vi "pulse length and delay.vi"() -> ()   [LabVIEW 2012]
uses:
  <vilib>/Analysis/NI_AALPro.lvlib
  <vilib>/Analysis/NI_AALBase.lvlib
panel:
  in  "index":i32=625
  out "Sigma":dbl format="%#_3p"
  out "Ch3 Err":dbl format="%_3p"
  out "Ch2 Err":dbl format="%_3p"
  out "Ch1 Err":dbl format="%_3p"
  out "Ch3 Mean":dbl format="%_3p"
  out "Ch2 Mean":dbl format="%_3p"
  out "Ch1 Mean":dbl format="%_3p"
  out "Mean":dbl format="%#_3p"
  in  "Measurement type":i32(ring) items=["Pulse Delay"=1, "Pulse Width"=0]
  out "Sum (%)":dbl format="%#_3g"
  in  "Fit":bool
  in  "Channel4 Threshold Voltage (mV)":i32
  out "Single Count Channel4":dbl format="%#_3p"
  out "Normal part R":dbl format="%#_3g"
  out "Normal part diff":dbl format="%#_3g"
  out "AP part":dbl format="%#_3g"
  out "Normal part Int":dbl format="%#_3f"
  out "Countrate":dbl format="%#_3p"
  out "amplitude":dbl format="%#_3p"
  out "Countrate dinamics":cluster{dbl, dbl, dbl}(graph)
  in  "Histogram Start 1 (ns)":i32=16
  in  "number":i32(ring) items=["Channel3"=2, "Channel2"=1, "Channel1"=0]
  out "Single Count Channel3":dbl format="%#_3p"
  out "Single Count Channel2":dbl format="%#_3p"
  in  "i last":i32
  in  "Reset 1":bool
  in  "Histogram Bin":string(combo)="0"
  out "Waveform Graph 1":cluster{dbl, dbl, dbl[][]}(graph) caption="Waveform Graph"
  out "Single Count Channel1":dbl format="%#_3p"
  out "Exposition time (ms)":i64
  out "Measurement index":i64
  out "Start OK":bool
  in  "Exit":bool
  in  "Channel3 Threshold Voltage (mV)":i32
  in  "Channel2 Threshold Voltage (mV)":i32
  in  "Channel1 Threshold Voltage (mV)":i32 min=0 max=5000 step=10
  in  "Exposition Time (ms)":i64
  # "Current"
  # "Mean"
  # "Err"
  # "Ch1"
  # "Ch2"
  # "Ch3"
  # "Ch4"
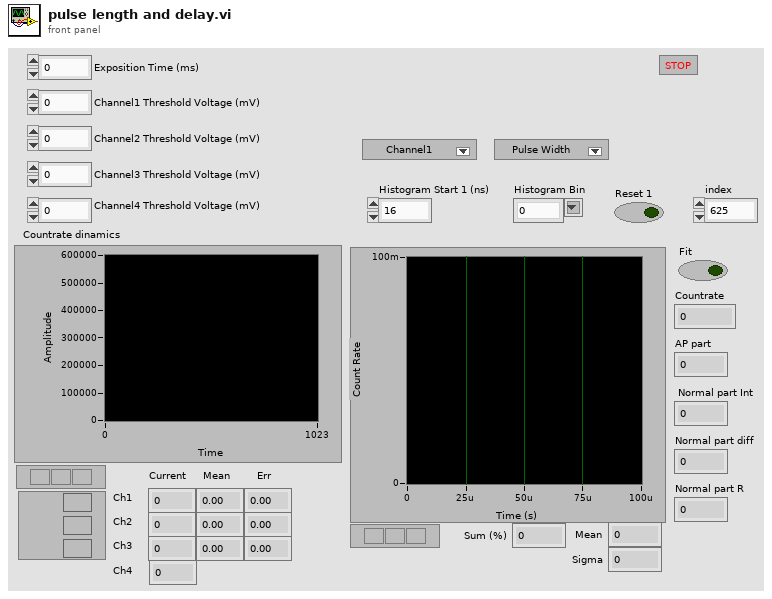
[diagram p1: front panel]
types:
  T1 = cluster{"Channel1":bool, "Channel2":bool, "Channel3":bool, "Channel4":bool}
  T2 = cluster{"[0]":i64, "Channel1 Threshold Voltage (mV)":i32, "Channel1 Pulse Front":string, "Channel2 Threshold Voltage (mV)":i32, "Channel2 Pulse Front":string, "Channel3 Threshold Voltage (mV)":i32, "Channel3 Pulse Front ":string, "Channel4 Threshold Voltage (mV)":i32, "Channel4 Pulse Front ":string, "Single Count Enable":cluster{"Channel1":bool, "Channel2":bool, "Channel3":bool, "Channel4":bool}, "Single Count Max":i32, "Sum Count Enable":cluster{"Channel1":bool, "Channel2":bool, "Channel3":bool, "Channel4":bool}, "Sum Count Max":i32, "Start-Stop1 Multyplex":cluster{"Stop Channel":string, "Start Channel":string}, "Stop Delay 1 (ns)":i16, "Window Length 1 (ns)":i32, "Window Offset 1 (ns) ":i32, "Conditional Correlation 1":string, "Histogram Bin 1":string, "Histogram Start 1 (ns) ":i32, "Start-Stop2 Multyplex ":cluster{"Stop Channel":string, "Start Channel":string}, "Stop Delay 2 (ns)":i16, "Window Length 2 (ns) ":i32, "Window Offset 2 (ns) ":i32, "Conditional Correlation 2":string, "Histogram Bin 2":string, "Histogram Start 2 (ns)  ":i32, "Start-Stop3 Multyplex":cluster{"Stop Channel":string, "Start Channel":string}, "Stop Delay 3 (ns)":i16, "Window Length 3 (ns) ":i32, "Window Offset 3 (ns) ":i32, "Conditional Correlation 3":string, "Histogram Bin 3":string, "Histogram Start 3 (ns) ":i32, "Start-Stop4 Multyplex":cluster{"Stop Channel":string, "Start Channel":string}, "Stop Delay 4 (ns)":i16, "Window Length 4 (ns)  ":i32, "Window Offset 4 (ns) ":i32, "Conditional Correlation 4":string, "Histogram Bin 4":string, "Histogram Start 4 (ns)  ":i32, "Coincidence Count Enable":cluster{"Start-Stop1":bool, "Start-Stop2":bool, "Start-Stop3":bool, "Start-Stop4":bool}, "Coincidence Count Max":i32, "Coincidence Sum Enable":cluster{"Start-Stop1":bool, "Start-Stop2":bool, "Start-Stop3":bool, "Start-Stop4":bool}, "Coincidence Sum Max":i32, "Output Channel Enable":cluster{"Channel1":bool, "Channel2":bool, "Channel3":bool, "Channel4":bool}, "Output Channel Inversion":cluster{"Channel1":bool, "Channel2":bool, "Channel3":bool, "Channel4":bool, "Output":bool}}
  T3 = cluster{"Going":bool, "Iinterrupted":bool, "Timer stop":bool, "Single count stop Ch1":bool, "Single count stop Ch2":bool, "Single count stop Ch3":bool, "Single count stop Ch4":bool, "Sum count stop":bool, "Coincidence count stop SS1":bool, "Coincidence count stop SS2":bool, "Coincidence count stop SS3":bool, "Coincidence count stop SS4":bool, "Coincidence sum count stop":bool, "Reserved":bool, "Correlator is not initialised":bool, "Internal error":bool}
  T4 = cluster{"Measurement index":i64, "Exposition time (ms)":i64, "Single Count Channel1":i64, "Single Count Channel2":i64, "Single Count Channel3":i64, "Single Count Channel4":i64, "Sum Single Count":i64, "Coincidence Count SS1":i64, "Coincidence Count SS2":i64, "Coincidence Count SS4":i64, "Coincidence Count SS5":i64, "Sum Coincidence Count":i64}
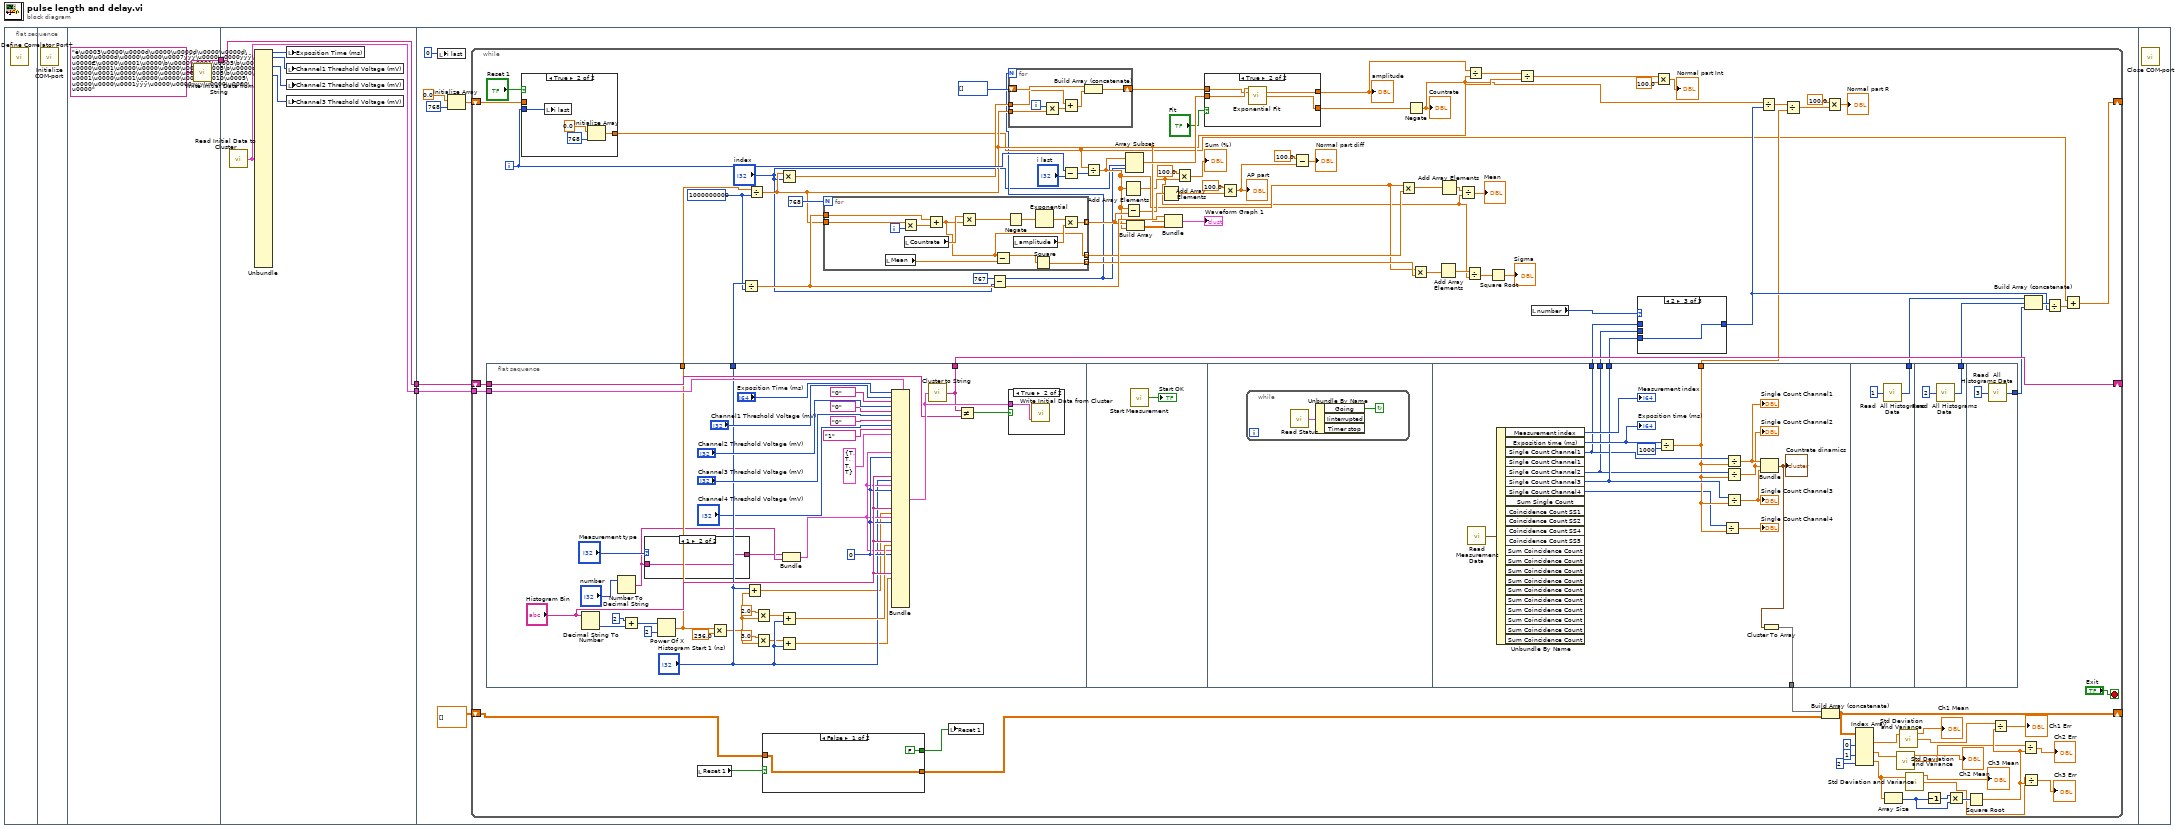
[diagram p0: block diagram]
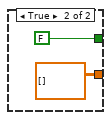
[diagram p2: hidden frame]
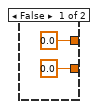
[diagram p3: hidden frame]
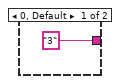
[diagram p7: hidden frame]
diagram:
  n1 = flat-sequence {
    tunnel: [w4] -> w1
    tunnel: [w10] -> w3
    tunnel: [w5] -> w2
    tunnel: w1 -> [w5]
    tunnel: w3 -> [w17]
    tunnel: w2 -> [w13]
    frame #0 {
      n2 = call "Define Correlator Port+.vi"() -> ()  [unwired: 3 in]
    }
    frame #1 {
      n3 = call "Initialize COM-port.vi"() -> ()  [unwired: 4 in]
    }
    frame #2 {
      w4 = "è\u0003\u0000\u0000d\u0000\u0000d\u0000\u0000d\u0000\u0000d\u0000\u0000\u0007ÿÿÿ\u0000\u0000ÿÿÿ\u0000€\u0000\u0001\u0000\b\u0000\u0001\u0005\b\u0000‘\u0000\u0001\u0000\u0000\u0000\u0002\u0005\b\u0000¢\u0000\u0001\u0000\u0000\u0000\u0004\u0005\b\u0000\u0001\u0000\u0001\u0000\u0000\u0000\u0010\u0005\u0000\u0000\u0001ÿÿÿ\u0000\u0000ÿÿÿ\u0000\u0000\u0000" ("string")
      n4 = call "Write Initial Data from String.vi"("Data"=w4) -> ()  [unwired: 1 out]
    }
    frame #3 {
      n5 = call "Read Initial Data to Cluster.vi"() -> ("Correlator Initial Data 2"=w10:T2)  [unwired: 2 in]
      n6 = Unbundle(w10) -> ("[0]"=w9:i64, "Channel1 Threshold Voltage (mV)"=w8:i32, "Channel2 Threshold Voltage (mV)"=w7:i32, "Channel3 Threshold Voltage (mV)"=w6:i32)  [unwired: 43 out]
      n7 = local write "Exposition Time (ms)"(w9) -> ()
      n8 = local write "Channel1 Threshold Voltage (mV)"(w8) -> ()
      n9 = local write "Channel2 Threshold Voltage (mV)"(w7) -> ()
      n10 = local write "Channel3 Threshold Voltage (mV)"(w6) -> ()
    }
    frame #4 {
      n11 = local write "i last"(0 ("i last")) -> ()
      n12 = Initialize Array(0.0 ("element"), 768 ("dimension size")) -> (w14:dbl[])
      n13 = while {
        tunnel: w17 -> [w110]
        shift-right: [w104] -> _
        shift-left: w14 -> [w102]
        shift-right: [w108] -> _
        shift-left: w13 -> [w107]
        shift-right: [w50] -> _
        shift-left: dbl[][] [] -> [w40]
        i -> [w100]
        stop <- "Exit" stop-if-true
        w105 = 1000000000 ("y")
        n14 = flat-sequence {
          tunnel: w110 -> [w182]
          tunnel: ["Histogram Start 1 (ns)"] -> w106
          tunnel: [w175] -> w108
          tunnel: w107 -> [w177]
          tunnel: [w167] -> w88
          tunnel: [w202] -> w91
          tunnel: [w204] -> w90
          tunnel: [w203] -> w92
          tunnel: [w197] -> w63
          tunnel: [w194] -> w51
          tunnel: [w209] -> w97
          tunnel: [w211] -> w95
          tunnel: [w213] -> w94
          frame #0 {
            w165 = i16 0 ("Stop Delay1  (ns)")
            n15 = Decimal String To Number(string="Histogram Bin") -> (number=w173:i32)  [unwired: 2 in, 1 out]
            n16 = Number To Decimal String(number="number") -> (decimal integer string=w152:string)  [unwired: 1 in]
            n17 = Add(x=2, y=w173) -> (x+y=w172:i32)
            n18 = case shown="1" "Measurement type" {
              tunnel: w152 -> [_ w189]
              tunnel: ["3" ("decimal integer string") w189] -> w151
              frame 0, Default {
              }
              frame 1 {
              }
            }
            n19 = Power Of X(1:i8 2 ("x"), 2:w172) -> (0:w167:dbl)
            n20 = Multiply(x=w167, y=256.0) -> (x*y=w161:dbl)
            n21 = Add(x="Histogram Start 1 (ns)", y=w161) -> (x+y=w156:dbl)
            n22 = Multiply(x=2.0, y=w161) -> (x*y=w160:dbl)
            n23 = Multiply(x=3.0, y=w161) -> (x*y=w158:dbl)
            n24 = Add(x=w160, y="Histogram Start 1 (ns)") -> (x+y=w168:dbl)
            n25 = Add(x=w158, y="Histogram Start 1 (ns)") -> (x+y=w162:dbl)
            n26 = Bundle("decimal integer string"=w151, w152) -> (w164:cluster{"decimal integer string":string, string})  [unwired: 1 in]
            n27 = Bundle(cluster=w182, "[0]"="Exposition Time (ms)", "Channel1 Threshold Voltage (mV)"="Channel1 Threshold Voltage (mV)", "Channel1 Pulse Front"="0", "Channel2 Threshold Voltage (mV)"="Channel2 Threshold Voltage (mV)", "Channel2 Pulse Front"="0", "Channel3 Threshold Voltage (mV)"="Channel3 Threshold Voltage (mV)", "Channel3 Pulse Front"="0", "Channel4 Threshold Voltage (mV)"="Channel4 Threshold Voltage (mV)", "Channel4 Pulse Front"="1" ("Channel2 Pulse Front"), "Single Count Enable"=T1 {"Channel1"=TRUE, "Channel2"=TRUE, "Channel3"=TRUE, "Channel4"=TRUE}, "Start-Stop1 Multyplex"=w164, "Stop Delay 1 (ns)"=w165, "Histogram Bin 1"="Histogram Bin", "Histogram Start 1 (ns)"="Histogram Start 1 (ns)", "Start-Stop2 Multyplex"=w164, "Stop Delay 2 (ns)"=w165, "Histogram Bin 2"="Histogram Bin", "Histogram Start 2 (ns)"=w156, "Start-Stop3 Multyplex"=w164, "Stop Delay 3 (ns)"=w165, "Histogram Bin 3"="Histogram Bin", "Histogram Start 3 (ns)"=w168, "Start-Stop4 Multyplex"=w164, "Stop Delay 4 (ns)"=w165, "Histogram Bin 4"="Histogram Bin", "Histogram Start 4 (ns)"=w162) -> (w178:T2)  [unwired: 21 in]
            n28 = call "Cluster to String.vi"("Correlator Initial Data"=w178) -> ("string"=w175:string)
            n29 = Not Equal?(x=w175, y=w177) -> (x != y?=w176:bool)
            n30 = case shown="True" w176 {
              tunnel: w178 -> [_ w190]
              frame False {
              }
              frame True {
                n31 = call "Write Initial Data from Cluster.vi"("Correlator Initial Data"=w190) -> ()  [unwired: 2 in, 1 out]
              }
            }
          }
          frame #1 {
            n32 = call "Start Measurement.vi"() -> ("Start OK"=→"Start OK":bool)  [unwired: 2 in]
          }
          frame #2 {
            n33 = while {
              stop <- w192 continue-if-true
              n34 = call "Read Status.vi"() -> ("Status Data"=w193:T3)  [unwired: 2 in]
              n35 = Unbundle By Name(w193) -> ("Going"=w192:bool)  [unwired: 2 out]
            }
          }
          frame #3 {
            n36 = call "Read Measurement Data.vi"() -> ("Measurement Data"=w207:T4)  [unwired: 3 in]
            n37 = Unbundle By Name(w207) -> ("Measurement index"=→"Measurement index":i64, "Exposition time (ms)"=w206:i64, "Single Count Channel1"=w203:i64, "Single Count Channel2"=w202:i64, "Single Count Channel3"=w204:i64, "Single Count Channel4"=w196:i64)  [unwired: 16 out]
            "Exposition time (ms)" <- w206
            n38 = Divide(x=w206, y=1000) -> (x/y=w197:dbl)
            n39 = Divide(x=w196, y=w197) -> (x/y=→"Single Count Channel4":dbl)
            n40 = Divide(x=w203, y=w197) -> (x/y=w201:dbl)
            "Single Count Channel1" <- w201
            n41 = Divide(x=w202, y=w197) -> (x/y=w200:dbl)
            "Single Count Channel2" <- w200
            n42 = Divide(x=w204, y=w197) -> (x/y=w199:dbl)
            "Single Count Channel3" <- w199
            n43 = Bundle(w201, w200, w199) -> (w195:cluster{dbl, dbl, dbl})  [unwired: 1 in]
            "Countrate dinamics" <- w195
            n44 = Cluster To Array(cluster=w195) -> (array=w194:dbl[])
          }
          frame #4 {
            n45 = call "Read  All Histograms Data.vi"("Start-Stop#"=i8 1) -> ("Array"=w209:i64[])
          }
          frame #5 {
            n46 = call "Read  All Histograms Data.vi"("Start-Stop#"=i8 2) -> ("Array"=w211:i64[])
          }
          frame #6 {
            n47 = call "Read  All Histograms Data.vi"("Start-Stop#"=i8 3) -> ("Array"=w213:i64[])
          }
        }
        n48 = case shown="True" "Reset 1" {
          tunnel: w102 -> [w146 _]
          tunnel: [w146 w147] -> w56
          tunnel: w100 -> [_ w148]
          frame False {
          }
          frame True {
            n49 = local write "i last"(w148) -> ()
            n50 = Initialize Array(0.0 ("element"), 768 ("dimension size")) -> (w147:dbl[])
          }
        }
        n51 = local read "Reset 1"() -> (w41:bool)
        n52 = Divide(x=w106, y=w105) -> (x/y=w76:dbl)
        n53 = Divide(x=w88, y=w105) -> (x/y=w75:dbl)
        n54 = case shown="False" w41 {
          tunnel: [w113 dbl[][] []] -> w39
          tunnel: w40 -> [w113 _]
          tunnel: [FALSE ("Reset") FALSE ("Reset")] -> w20
          frame False {
          }
          frame True {
          }
        }
        n55 = Multiply(x=w75, y="index") -> (x*y=w86:dbl)
        n56 = for {
          N: 768 -> [_]
          tunnel: w76 -> [w135]
          tunnel: w75 -> [w133]
          tunnel: [w127] -> w73 mode=indexing
          tunnel: [w123] -> w55 mode=indexing
          tunnel: [w125] -> w27 mode=indexing
          i -> [w134]
          n57 = local read "Mean"() -> (w124:dbl)
          n58 = Multiply(x=w133, y=w134) -> (x*y=w132:dbl)
          n59 = local read "Countrate"() -> (w131:dbl)
          n60 = Add(x=w135, y=w132) -> (x+y=w123:dbl)
          n61 = Multiply(x=w131, y=w123) -> (x*y=w130:dbl)
          n62 = Subtract(x=w123, y=w124) -> (x-y=w122:dbl)
          n63 = Negate(x=w130) -> (-x=w126:dbl)
          n64 = local read "amplitude"() -> (w128:dbl)
          n65 = Square(x=w122) -> (x^2=w125:dbl)
          n66 = Exponential(1:w126) -> (0:w129:dbl)
          n67 = Multiply(x=w129, y=w128) -> (x*y=w127:dbl)
        }
        n68 = local write "Reset 1"(w20) -> ()
        n69 = Subtract(x=767 ("length"), y="index") -> (x-y=w19:i32)
        n70 = for {
          N: w19 -> [_]
          tunnel: w86 -> [w138]
          shift-right: [w141] -> w78
          shift-left: i32[] [] -> [w139]
          tunnel: w75 -> [w136]
          i -> [w142]
          n71 = Multiply(x=w142, y=w136) -> (x*y=w137:dbl)
          n72 = Add(x=w138, y=w137) -> (x+y=w140:dbl)
          n73 = Build Array (concatenate)(w139, w140) -> (w141:dbl[])
        }
        n74 = Subtract(x=w100, y="i last") -> (x-y=w98:i32)
        n75 = Divide(x=w56, y=w98) -> (x/y=w26:dbl[])
        n76 = Add Array Elements(numeric array=w26) -> (sum=w23:dbl)
        n77 = Subtract(x=w26, y=w73) -> (x-y=w72:dbl[])
        n78 = Array Subset(array=w26, index="index", length=w19) -> (w79:dbl[])
        n79 = Build Array(w73, w26) -> (w74:dbl[][])
        n80 = Add Array Elements(numeric array=w72) -> (sum=w71:dbl)
        n81 = Bundle(w76, w75, w74) -> (→"Waveform Graph 1":cluster{dbl, dbl, dbl[][]})  [unwired: 1 in]
        n82 = Multiply(x=100.0, y=w23) -> (x*y=→"Sum (%)":dbl)
        n83 = case shown="True" "Fit" {
          tunnel: [0.0 ("damping") w121] -> w85
          tunnel: [0.0 ("amplitude") w120] -> w82
          tunnel: w79 -> [_ w119]
          tunnel: w78 -> [_ w118]
          frame False {
          }
          frame True {
            n84 = call <vilib>:"Exponential Fit.vi"("Y"=w119, "X"=w118) -> ("amplitude"=w120:dbl, "damping"=w121:dbl)  [unwired: 8 in, 4 out]
          }
        }
        "amplitude" <- w82
        n85 = Multiply(x=100.0, y=w71) -> (x*y=w69:dbl)
        "AP part" <- w69
        n86 = Subtract(x=100.0, y=w69) -> (x-y=→"Normal part diff":dbl)
        n87 = Multiply(x=w26, y=w55) -> (x*y=w54:dbl[])
        n88 = Negate(x=w85) -> (-x=w66:dbl)
        "Countrate" <- w66
        n89 = Multiply(x=w26, y=w27) -> (x*y=w25:dbl[])
        n90 = Add Array Elements(numeric array=w25) -> (sum=w24:dbl)
        n91 = Add Array Elements(numeric array=w54) -> (sum=w53:dbl)
        n92 = Divide(x=w53, y=w23) -> (x/y=→"Mean":dbl)
        n93 = Divide(x=w24, y=w23) -> (x/y=w22:dbl)
        n94 = Divide(x=w82, y=w66) -> (x/y=w84:dbl)
        n95 = Square Root(x=w22) -> (sqrt(x)=→"Sigma":dbl)
        n96 = Divide(x=w84, y=w75) -> (x/y=w83:dbl)
        n97 = local read "number"() -> (w93:i32)
        n98 = case shown="2" w93 {
          tunnel: [w143 w144 w145] -> w65
          tunnel: w92 -> [w143 _ _]
          tunnel: w91 -> [_ w144 _]
          tunnel: w90 -> [_ _ w145]
          frame 0, Default {
          }
          frame 1 {
          }
          frame 2 {
          }
        }
        n99 = Multiply(x=w83, y=100.0) -> (x*y=→"Normal part Int":dbl)
        n100 = Divide(x=w66, y=w65) -> (x/y=w64:dbl)
        n101 = Divide(x=w64, y=w63) -> (x/y=w62:dbl)
        n102 = Build Array (concatenate)(w51, w39) -> (w50:dbl[][])
        n103 = Multiply(x=100.0, y=w62) -> (x*y=→"Normal part R":dbl)
        n104 = Index Array(array=w50, index (col) #1=0 ("disabled index (col)"), index (col) #2=1 ("index (col)"), index (col) #3=2 ("index (col)")) -> (element #1=w46:dbl[], element #2=w45:dbl[], element #3=w38:dbl[])  [unwired: 3 in]
        n105 = Array Size(array=w38) -> (size(s)=w36:i32)
        n106 = call <vilib>:"Std Deviation and Variance.vi"("X"=w45) -> ("mean"=→"Ch2 Mean":dbl, "standard deviation"=w32:dbl)  [unwired: 1 in, 1 out]
        n107 = call <vilib>:"Std Deviation and Variance.vi"("X"=w46) -> ("mean"=→"Ch1 Mean":dbl, "standard deviation"=w33:dbl)  [unwired: 1 in, 1 out]
        n108 = call <vilib>:"Std Deviation and Variance.vi"("X"=w38) -> ("mean"=→"Ch3 Mean":dbl, "standard deviation"=w31:dbl)  [unwired: 1 in, 1 out]
        n109 = Decrement(x=w36) -> (x-1=w37:i32)
        n110 = Multiply(x=w37, y=w36) -> (x*y=w35:i32)
        n111 = Square Root(x=w35) -> (sqrt(x)=w34:dbl)
        n112 = Divide(x=w33, y=w34) -> (x/y=→"Ch1 Err":dbl)
        n113 = Divide(x=w32, y=w34) -> (x/y=→"Ch2 Err":dbl)
        n114 = Divide(x=w31, y=w34) -> (x/y=→"Ch3 Err":dbl)
        n115 = Build Array (concatenate)(w97, w95, w94) -> (w96:i64[])
        n116 = Divide(x=w96, y=w65) -> (x/y=w103:dbl[])
        n117 = Add(x=w56, y=w103) -> (x+y=w104:dbl[])
      }
    }
    frame #5 {
      n118 = call "Close COM-port.vi"() -> ()  [unwired: 4 in]
    }
  }
